vi "T_dual.vi"(2 "S":bool, 3 "C":bool, 4 "D":bool, 5 "R":bool) -> (0 "NOT Q":bool, 1 "Q":bool)   [LabVIEW 2013]
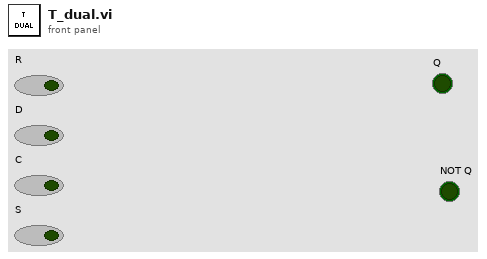
[diagram p1: front panel]
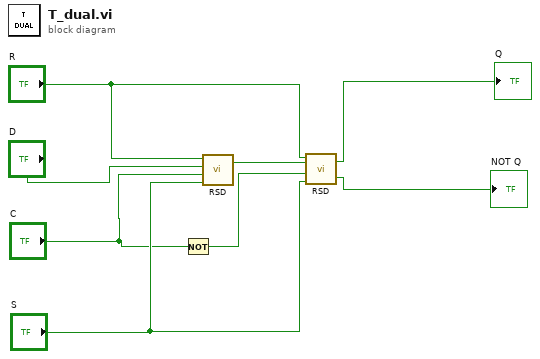
[diagram p0: block diagram]
diagram:
  n1 = Not(x="C") -> (.not. x?=w5:bool)
  n2 = call "RSD.vi"("S"="S", "C"="C", "D"="D", "R"="R") -> ("Q1"=w3:bool)  [unwired: 1 out]
  n3 = call "RSD.vi"("S"="S", "C"=w5, "D"=w3, "R"="R") -> ("Q2"=→"NOT Q":bool, "Q1"=→"Q":bool)
